vi "RSZVB Get Other Sources State.vi"(8 "error in (no error)":errorcluster {"code" format="%.0x"}, 10 "Channel (1)":i32=1, 11 "VISA session":refnum<visa-resource-name>) -> (0 "error out":errorcluster {"code" format="%.0x"}, 2 "Other Sources":bool, 3 "dup VISA session":refnum<visa-resource-name>)   [LabVIEW 2011]
doc: "This VI returns the state of all other sources during the calibration sweep for channel <Ch>.\n\nRemote-control command(s):\nSOURce<Ch>:POWer<Pt>:CORRection:OSOurces[:STATe]?"
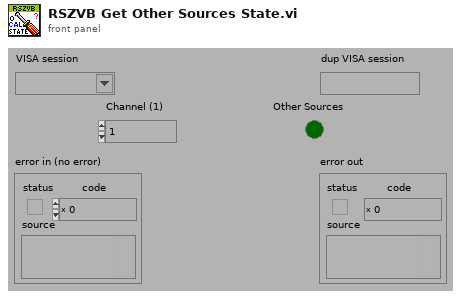
[diagram p1: front panel]
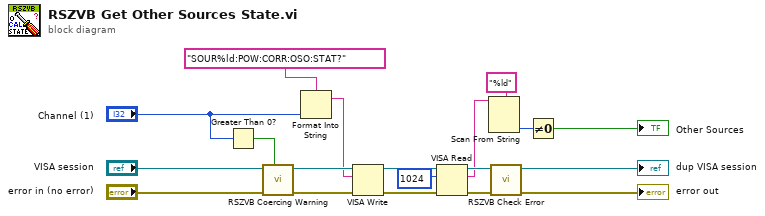
[diagram p0: block diagram]
diagram:
  n1 = Greater Than 0?(x="Channel (1)") -> (x > 0?=w7:bool)
  n2 = call "RSZVB Coercing Warning.vi"("In Range?"=w7, "error in (no error)"="error in (no error)", "VISA session"="VISA session") -> ("error out"=w17:errorcluster, "dup VISA session"=w18:refnum<visa-resource-name>)  [unwired: 7 in]
  n3 = Format Into String(format string="SOUR%ld:POW:CORR:OSO:STAT?", "Channel (1)") -> (resulting string=w16:string)  [unwired: 2 in, 1 out]
  n4 = VISA Write(VISA resource name=w18, write buffer=w16, error in (no error)=w17) -> (VISA resource name out=w9:refnum<visa-resource-name>, error out=w8:errorcluster)  [unwired: 1 out]
  n5 = VISA Read(VISA resource name=w9, byte count=u32 1024 ("byte count (0)"), error in (no error)=w8) -> (VISA resource name out=w14:refnum<visa-resource-name>, read buffer=w11:string, error out=w13:errorcluster)  [unwired: 1 out]
  n6 = Scan From String(format string="%ld", input string=w11) -> (output 1=w10:i32)  [unwired: 3 in, 3 out]
  n7 = call "RSZVB Check Error.vi"("error in (no error)"=w13, "VISA session"=w14) -> ("error out"=→"error out":errorcluster, "dup VISA session"=→"dup VISA session":refnum<visa-resource-name>)  [unwired: 8 in]
  n8 = Not Equal To 0?(x=w10) -> (x != 0?=→"Other Sources":bool)
